vi "Pcre2GetMatchResult8.vi"(8 "error in":errorcluster, 11 "pMatchData":u64 format="%.0x") -> (0 "error out":errorcluster, 2 "MatchResult":i32, 3 "pMatchData":u64 format="%.0x")   [LabVIEW 2021, in "libpcre2-8.lvlib"]
uses:
  libpcre2-8.lvlib
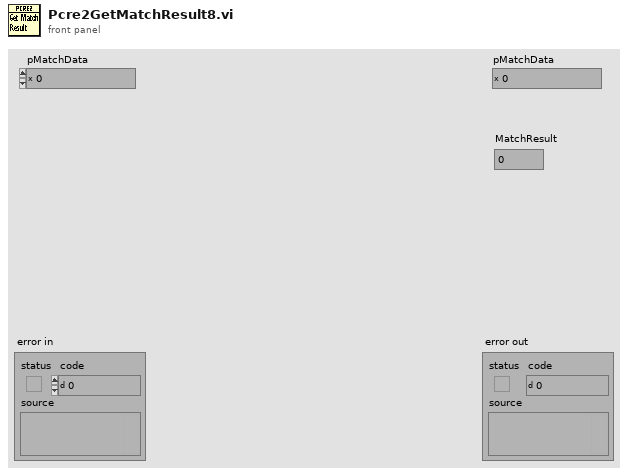
[diagram p1: front panel]
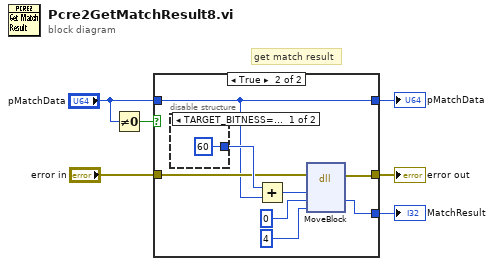
[diagram p0: block diagram]
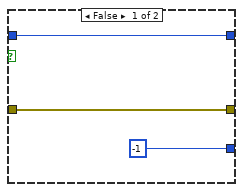
[diagram p2: hidden frame]
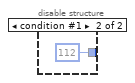
[diagram p3: hidden frame]
diagram:
  # "get match result"
  n1 = Not Equal To 0?(x="pMatchData") -> (x != 0?=w2:bool)
  n2 = case shown="True" w2 {
    tunnel: "error in" -> [w9 w13]
    tunnel: [w8 w11] -> w5
    tunnel: [w9 w12] -> w4
    tunnel: [-1 ("pointerDest") w10] -> w1
    tunnel: "pMatchData" -> [w8 w11]
    frame False {
    }
    frame True {
      n3 = disable-structure shown="TARGET_BITNESS==32, Default" {
        disable-tunnel: [u64 60 u64 112] -> w16
        frame condition #0 (active) {
        }
        frame condition #1 {
        }
      }
      n4 = Add(x=w16, y=w11) -> (x+y=w17:u64)
      n5 = dll-call lib="LabVIEW" fn="MoveBlock"(error in=w13, "pointerSrc"=w17, "pointerDest"=0 ("size"), "size"=u64 4) -> (error out=w12:errorcluster, "pointerDest"=w10:i32)  [unwired: 5 in, 1 out]
    }
  }
  "pMatchData" <- w5
  "error out" <- w4
  "MatchResult" <- w1
